vi "LCD Command.vi"() -> ()   [LabVIEW 2017, in "HD44780 FPGA.lvlib"]
uses:
  HD44780 FPGA.lvlib
panel:
  in  "LCD Command":T1={"device index (-1)"=-1, "operation (0)"=0}
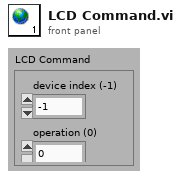
[diagram p1: front panel]
types:
  T1 = cluster{"device index (-1)":i8, "operation (0)":u32}
diagram:
